vi "NI VeriStand - Show Progress Dialog.vi"(8 "error in (no error)":errorcluster) -> (0 "error out":errorcluster)   [LabVIEW 2020, in "Custom Device API.lvlib"]
uses:
  <vilib>/NI VeriStand/Custom Device API/Custom Device API.lvlib
  98412ee5-b41a-48c7-884c-835b087eb80e.vi
  <vilib>/NI VeriStand/Custom Device API/Custom Device Offline Path.vi
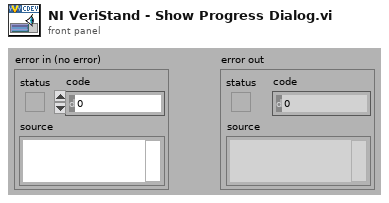
[diagram p1: front panel]
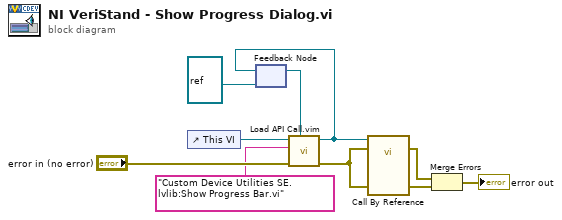
[diagram p0: block diagram]
diagram:
  n1 = control-ref of="This VI"() -> (w7:refnum<vi>)
  n2 = feedback #1(refnum<vi> refnum ("type specifier VI Refnum (for type only)")) -> (w8:refnum<vi>)
  n3 = call "Load API Call.vim"("VI reference in"=w8, "error in (no error)"="error in (no error)", "VI qualified name"="Custom Device Utilities SE.lvlib:Show Progress Bar.vi", "Caller VI ref"=w7) -> ("error out"=w4:errorcluster, "VI reference"=w5:refnum<vi>)  [unwired: 6 in]
  n4 = feedback-in #1(w5) -> ()
  n5 = call-by-ref "?"(reference=w5, error in=w4, 8:"error in (no error)"=w4) -> (error out=w1:errorcluster, 0:"error out"=w10:errorcluster)  [unwired: 10 in, 1 out]
  n6 = Merge Errors(w1, w10) -> (→"error out":errorcluster)
